vi "Robot Global Data.vi"() -> ()   [LabVIEW 2012]
doc: "This global VI can contain as many global variables as you need. Place a control on the panel, give it a good name. To read or write to it from a VI, drag the icon to the diagram of that VI. You can also drag from the project. Click on the node to change which global you access. You shouldn't have multiple locations writing to a global or it will cause a race-condition."
uses:
  <vilib>/Rock Robotics/WPI/DriverStation/WPI_DriverStationRobotMode2.ctl
panel:
  out "Dash Data":T1
  in  "Robot Mode":T2
  in  "LED toggle rate (ms)":u32=20
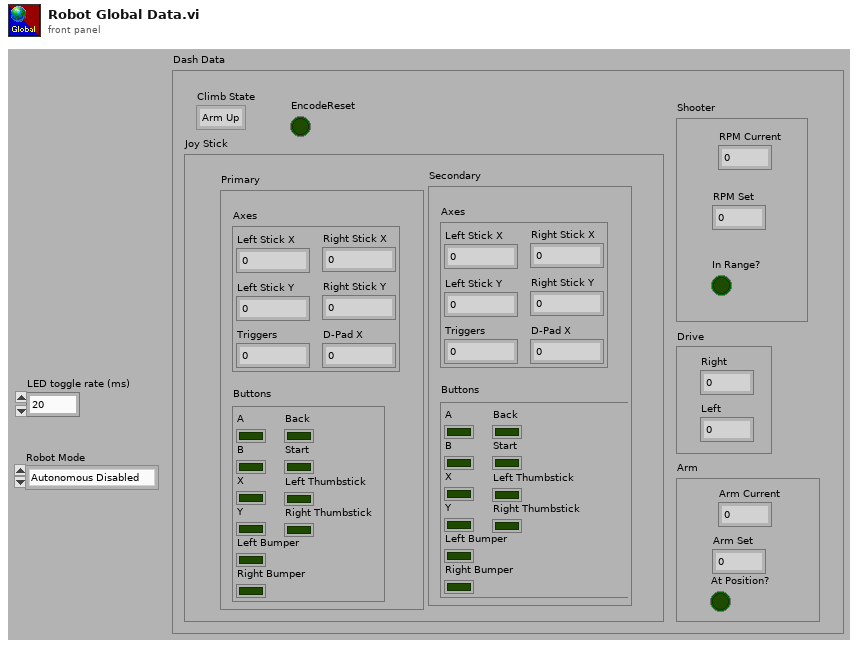
[diagram p1: front panel]
types:
  T1 = cluster{"Joy Stick":cluster{"Secondary":cluster{"Buttons":cluster{"A":bool, "B":bool, "X":bool, "Y":bool, "Left Bumper":bool, "Right Bumper":bool, "Back":bool, "Start":bool, "Left Thumbstick":bool, "Right Thumbstick":bool}, "Axes":cluster{"Left Stick X ":dbl, "Left Stick Y":dbl, "Triggers":dbl, "Right Stick X":dbl, "Right Stick Y":dbl, "D-Pad X":dbl}}, "Primary":cluster{"Buttons":cluster{"A":bool, "B":bool, "X":bool, "Y":bool, "Left Bumper":bool, "Right Bumper":bool, "Back":bool, "Start":bool, "Left Thumbstick":bool, "Right Thumbstick":bool}, "Axes":cluster{"Left Stick X ":dbl, "Left Stick Y":dbl, "Triggers":dbl, "Right Stick X":dbl, "Right Stick Y":dbl, "D-Pad X":dbl}}}, "Arm":cluster{"Arm Set":dbl, "Arm Current":dbl, "At Position?":bool}, "Drive":cluster{"Right":dbl, "Left":dbl}, "Shooter":cluster{"RPM Current":dbl, "RPM Set":dbl, "In Range?":bool}, "Climb State":enum16{"Arm Up", "Arm Down", "Arm Attach", "Arm Wait"}, "EncodeReset":bool}
  T2 = typedef "WPI_DriverStationRobotMode2.ctl" = enum16{"Autonomous Disabled", "Autonomous Enabled", "Teleop Disabled", "Teleop Enabled", "Timeout", "Finish", "Test Disabled", "Test Enabled"}
diagram:
